vi "uObserver_Publish_Events.vi"(8 "error in (no error)":errorcluster, 10 "uMsgs":refnum<class "uMsg.lvclass">[](array[class]), 11 "uObserver in":refnum<class "uObserver.lvclass">) -> (0 "error out":errorcluster, 3 "uObserver out":refnum<class "uObserver.lvclass">)   [LabVIEW 2023, in "uFramework_pack_uActor.lvlib" / "uObserver.lvclass"]
doc: "Publish a batch of eventsto the observed broker conforming to the Observer's publishing policy."
uses:
  uObserver.lvclass
  Bin/uFramework.lvlibp/uMsg/uMsg.lvclass
  uObserver.lvclass/uObserver.ctl
  Bin/uFramework.lvlibp/uClient_Publisher/uClient_Publisher.lvclass
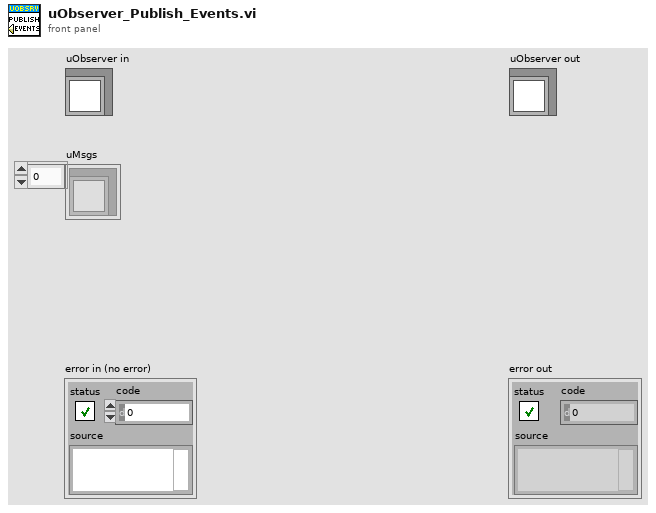
[diagram p1: front panel]
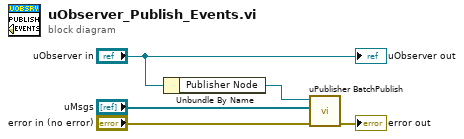
[diagram p0: block diagram]
diagram:
  n1 = Unbundle By Name("uObserver in") -> ("Publisher Node"=w1:refnum<class "uClient_Publisher.lvclass">)
  n2 = call "uPublisher BatchPublish.vi"("error in (no error)"="error in (no error)", "uMsgs"="uMsgs", "uClient_Publisher in"=w1) -> ("error out"=→"error out":errorcluster)  [unwired: 7 in, 1 out]
  "uObserver out" <- "uObserver in"
